vi "点对应单元格位置.vi"(8 "错误输入（无错误）":errorcluster, 10 "点":T2 caption="表格点", 11 "引用":refnum<vi>) -> (0 "错误输出":errorcluster, 2 "单元格大小":T1, 3 "引用输出":refnum<vi>)   [LabVIEW 2014, in "表格.lvlib"]
uses:
  <vilib>/Utility/miscctls.llb/LVPositionTypeDef.ctl
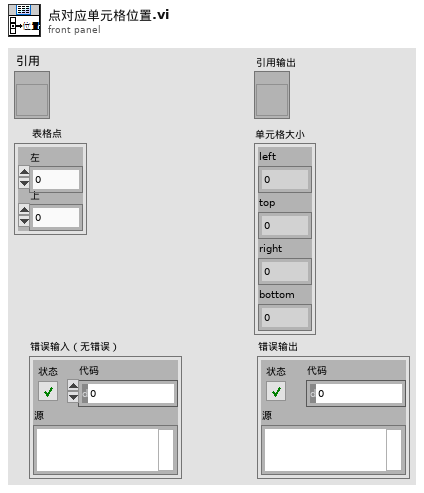
[diagram p1: front panel]
types:
  T1 = cluster{"left":i16, "top":i16, "right":i16, "bottom":i16}
  T2 = typedef "LVPositionTypeDef.ctl" = cluster{"Left":i32, "Top":i32}
  T3 = typedef "LVRowAndColumnTypeDef.ctl" = cluster{"Row":i32, "Column":i32}
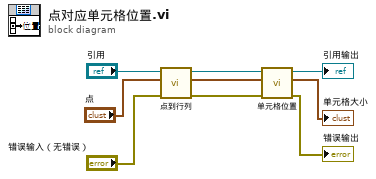
[diagram p0: block diagram]
diagram:
  n1 = call "点到行列.vi"("错误输入（无错误）"="错误输入（无错误）", "点"="点", "引用"="引用") -> ("错误输出"=w8:errorcluster, "单元格位置"=w9:T3, "引用输出"=w7:refnum<vi>)  [unwired: 6 in]
  n2 = call "单元格位置.vi"("错误输入（无错误）"=w8, "单元格位置"=w9, "Table输入"=w7) -> ("错误输出"=→"错误输出":errorcluster, "单元格大小"=→"单元格大小":T1, "Table输出"=→"引用输出":refnum<vi>)  [unwired: 6 in]
